vi "GFITS_postfix.vi"(9 "Database RefNum in":T1, 10 "imname in":string) -> (2 "imname out":string)   [LabVIEW 2016]
uses:
  DBSHAND/private/vis/DatabaseHand_RefNum.ctl
  DBSHAND/private/vis/DatabaseHand_Element_Get(string).vi
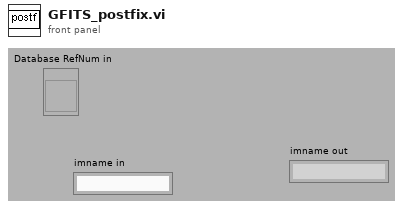
[diagram p1: front panel]
types:
  T1 = typedef "DatabaseHand_RefNum.ctl" = refnum<vi>
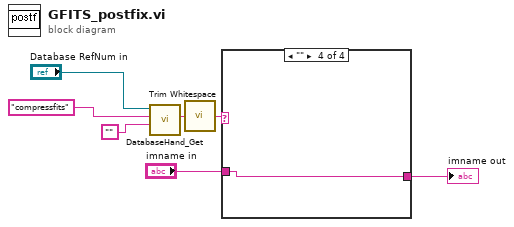
[diagram p0: block diagram]
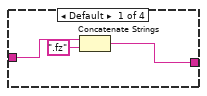
[diagram p2: hidden frame]
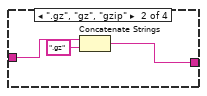
[diagram p3: hidden frame]
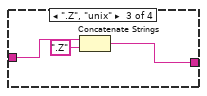
[diagram p4: hidden frame]
diagram:
  n1 = call-poly "DatabaseHand_Get.vi"("default value"="", "name"="compressfits", "Database RefNum in"="Database RefNum in") -> ("value"=w4:string)  [unwired: 2 in, 6 out]
  n2 = call <vilib>:"Trim Whitespace.vi"("string"=w4) -> ("trimmed string"=w1:string)  [unwired: 1 in]
  n3 = case shown="\"\"" w1 {
    tunnel: "imname in" -> [w10 w13 w16 w17]
    tunnel: [w9 w12 w15 w17] -> w2
    frame Default {
      n4 = Concatenate Strings(w10, ".fz" ("string")) -> (w9:string)
    }
    frame ".gz", "gz", "gzip" {
      n5 = Concatenate Strings(w13, ".gz" ("string")) -> (w12:string)
    }
    frame ".Z", "unix" {
      n6 = Concatenate Strings(w16, ".Z" ("string")) -> (w15:string)
    }
    frame "" {
    }
  }
  "imname out" <- w2
